vi "Configure Curve Point.vi"(0 "VISA resource name":refnum<visa-resource-name>, 1 "Temperature Value (0.0000)":dbl min=-9999.0 max=9999.0 step=1e-05 format="%.5f", 2 "Curvature Value (0.00000)":dbl min=-9999.9999 max=9999.9999 step=1e-06 format="%.5f", 5 "Curve (21)":i32=21 min=21 max=59 step=1, 7 "Index (1)":i32=1 min=1 max=200 step=1, 9 "Units Value (0.00000)":dbl min=-9999.0 max=9999.0 step=1e-05 format="%.5f", 11 "error in (no error)":errorcluster) -> (4 "VISA resource name out":refnum<visa-resource-name>, 15 "error out":errorcluster)   [LabVIEW 2015, in "Lake Shore 372.lvlib"]
doc: "Specifies the curve data point using <B>CRVPT</B>. The curvature value is only required for loading a cubic spline interpolation curve and is omitted when sending linear interpolation curves."
uses:
  <instrlib>/Lake Shore 372/Lake Shore 372.lvlib
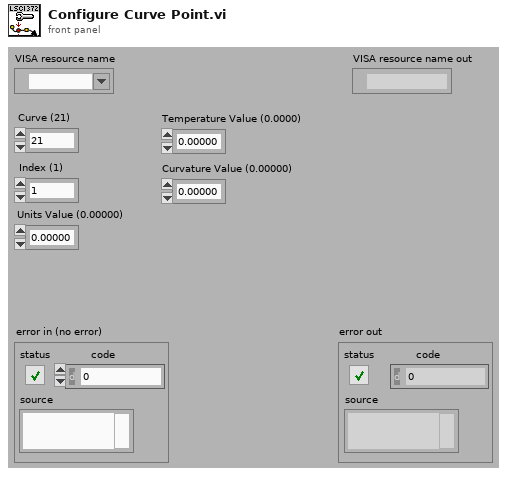
[diagram p1: front panel]
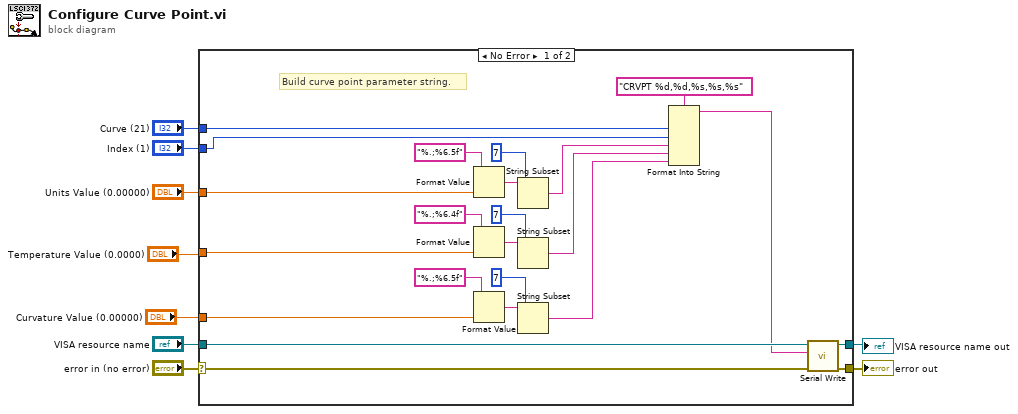
[diagram p0: block diagram]
diagram:
  n1 = case shown="No Error" "error in (no error)" {
    selector: "error in (no error)" -> [w16 w33]
    tunnel: "VISA resource name" -> [w28 w34]
    tunnel: [w27 w33] -> w8
    tunnel: [w26 w34] -> w7
    tunnel: "Curve (21)" -> [w14 _]
    tunnel: "Index (1)" -> [w13 _]
    tunnel: "Units Value (0.00000)" -> [w12 _]
    tunnel: "Temperature Value (0.0000)" -> [w11 _]
    tunnel: "Curvature Value (0.00000)" -> [w10 _]
    frame No Error {
      # "Build curve point parameter string."
      n2 = Format Value(format string="%.;%6.5f", value (0)=w12) -> (output string=w25:string)  [unwired: 1 in]
      n3 = Format Value(format string="%.;%6.4f", value (0)=w11) -> (output string=w24:string)  [unwired: 1 in]
      n4 = Format Value(format string="%.;%6.5f", value (0)=w10) -> (output string=w23:string)  [unwired: 1 in]
      n5 = String Subset(string=w25, length (rest)=7) -> (substring=w20:string)  [unwired: 1 in]
      n6 = String Subset(string=w24, length (rest)=7) -> (substring=w19:string)  [unwired: 1 in]
      n7 = String Subset(string=w23, length (rest)=7) -> (substring=w18:string)  [unwired: 1 in]
      n8 = Format Into String(format string="CRVPT %d,%d,%s,%s,%s", w14, w13, w20, w19, w18) -> (resulting string=w17:string)  [unwired: 2 in, 1 out]
      n9 = call <instrlib>:"Serial Write.vi"("error in (no error)"=w16, "Write Buffer (\"\")"=w17, "VISA resource name"=w28) -> ("error out"=w27:errorcluster, "VISA resource name out"=w26:refnum<visa-resource-name>)  [unwired: 6 in, 1 out]
    }
    frame Error {
    }
  }
  "error out" <- w8
  "VISA resource name out" <- w7
